vi "Set Switch Config by Package Type.vi"(5 "Package_Type":T1, 7 "Pins":string[](array[string])=["SW1", "SW2"], 8 "error in (no error)":errorcluster, 11 "Semiconductor Module Context":T2) -> (0 "error out":errorcluster)   [LabVIEW 2013]
uses:
  <vilib>/NI_TestStand_SemiconductorModule/NI_TestStand_Semiconductor_Module.lvlibp/PinMap/General/SemiconductorModuleContext.ctl
  Controls/Package_Type.ctl
  <vilib>/NI_TestStand_SemiconductorModule/NI_TestStand_Semiconductor_Module.lvlibp/PinMap/HSDIO/PinsToNIHSDIOSessions.vi
  <vilib>/NI_TestStand_SemiconductorModule/NI_TestStand_Semiconductor_Module.lvlibp
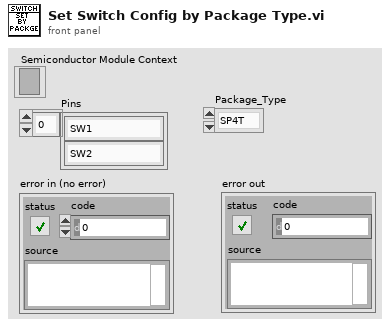
[diagram p1: front panel]
types:
  T1 = typedef "Package_Type.ctl" = enum16{"SP4T", "SP3T", "Sh3T", "Sh4T", "Guardian"}
  T2 = typedef "NI_TestStand_Semiconductor_Module.lvlibp/SemiconductorModuleContext.ctl" = refnum<k7>
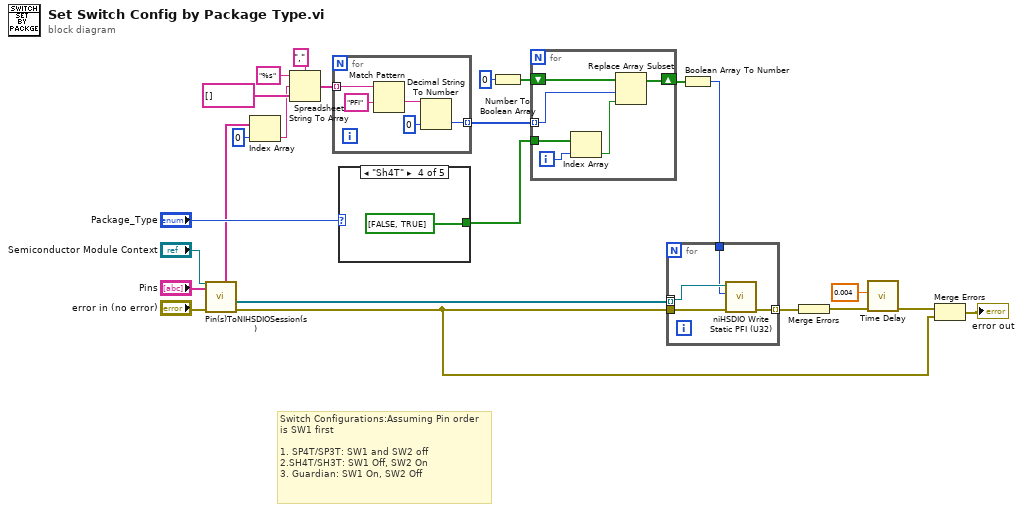
[diagram p0: block diagram]
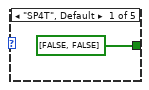
[diagram p2: hidden frame]
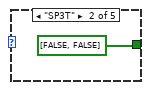
[diagram p3: hidden frame]
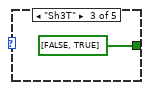
[diagram p4: hidden frame]
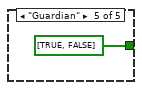
[diagram p5: hidden frame]
diagram:
  # "Switch Configurations:Assuming Pin order is SW1 first\n\n1. SP4T/SP3T: SW1 and SW2 off\n2.SH4T/SH3T: SW1 Off, SW2 On\n3. Guardian: SW1 On, SW2 Off"
  n1 = call-poly <vilib>:"Pin(s)ToNIHSDIOSession(s).vi"("error in (no error)"="error in (no error)", "Pins"="Pins", "Semiconductor Module Context"="Semiconductor Module Context") -> ("error out"=w13:errorcluster, "Generation Sessions"=w12:refnum<k15>[], "Channel Lists"=w1:string[])  [unwired: 3 in, 3 out]
  n2 = Index Array(array=w1, index=0) -> (element=w3:string)
  n3 = Spreadsheet String To Array(delimiter (Tab)=",", format string="%s", spreadsheet string=w3, array type (2D Dbl)=string[] []) -> (array=w2:string[])
  n4 = for {
    tunnel: w2 -> [w26] mode=indexing
    tunnel: [w25] -> w18 mode=indexing
    n5 = Match Pattern(string=w26, regular expression="PFI") -> (after substring=w29:string)  [unwired: 1 in, 3 out]
    n6 = Decimal String To Number(string=w29, default (0L)=0 ("default (0 I32)")) -> (number=w25:i32)  [unwired: 1 in, 1 out]
  }
  n7 = case shown="\"Sh4T\"" "Package_Type" {
    tunnel: [bool[] [FALSE, FALSE] bool[] [FALSE, FALSE] bool[] [FALSE, TRUE] bool[] [FALSE, TRUE] bool[] [TRUE, FALSE]] -> w14
    frame "SP4T", Default {
    }
    frame "SP3T" {
    }
    frame "Sh3T" {
    }
    frame "Sh4T" {
    }
    frame "Guardian" {
    }
  }
  n8 = Number To Boolean Array(number=0 ("Numeric")) -> (Boolean array=w17:bool[])
  n9 = for {
    tunnel: w18 -> [w37] mode=indexing
    shift-right: [w35] -> w16
    shift-left: w17 -> [w38]
    tunnel: w14 -> [w40]
    i -> [w39]
    n10 = Index Array(array=w40, index=w39) -> (element=w36:bool)
    n11 = Replace Array Subset(array=w38, new element=w36, index=w37) -> (w35:bool[])
  }
  n12 = Boolean Array To Number(Boolean array=w16) -> (number=w11:u32)
  n13 = for {
    tunnel: w13 -> [w44]
    tunnel: [w43] -> _ mode=indexing
    tunnel: w12 -> [w43] mode=indexing
    tunnel: w11 -> [w42]
    tunnel: [w41] -> w10 mode=indexing
    n14 = call <instrlib>:"niHSDIO Write Static PFI (U32).vi"("error in (no error)"=w44, "write data (0x0000)"=w42, "instrument handle"=w43) -> ("error out"=w41:errorcluster)  [unwired: 7 in, 1 out]
  }
  n15 = Merge Errors(w10) -> (w9:errorcluster)
  n16 = call "Time Delay"("error in (no error)"=w9, "Delay Time (s)"=0.004) -> ("error out"=w20:errorcluster)  [unwired: 9 in]
  n17 = Merge Errors(w20, w13) -> (→"error out":errorcluster)
